vi "Simple Reader.vi"(8 "error in (no error)":errorcluster, 11 "Ocean Optics Driver in":refnum<class "Ocean Optics Driver.lvclass">) -> (0 "error out":errorcluster, 2 "Signals":dbl[](array[numeric]), 3 "Ocean Optics Driver out":refnum<class "Ocean Optics Driver.lvclass">)   [LabVIEW 2016, in "Ocean Optics Driver.lvclass"]
uses:
  Ocean Optics Driver.lvclass
  C:/github/NHMFL_Core/Libraries/Instruments/Instrument Driver/Instrument Driver.lvclass
  C:/github/NHMFL_Core/Libraries/Instruments/Spectrometer Driver/Spectrometer Driver.lvclass
  Instrument Driver/Instrument Driver.lvclass/Instrument Driver.ctl
  Spectrometer Driver/Spectrometer Driver.lvclass/Spectrometer Driver.ctl
  Instrument Driver/Write Channel names.vi
  Instrument Driver/Write Channel units.vi
  Spectrometer Driver/Read Peaks.vi
  Read Ocean optics configuration.vi
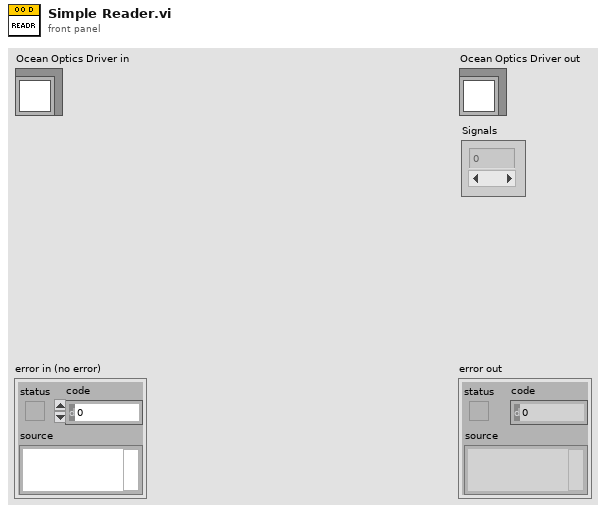
[diagram p1: front panel]
types:
  T1 = typedef "Peak Parameters.ctl" = cluster{"Amplitude":dbl, "Center":dbl, "Width":dbl}
  T2 = typedef "Ruby Spectra.lvclass/Ocean optics configuration.ctl" = cluster{"Integration time":dbl, "Fit parameters":T3, "Fit":bool, "Auto-update params":bool, "Save spectra":bool, "Reference wavelengh":dbl, "Background":path}
  T3 = typedef "Multi-peak Parameters.ctl" = cluster{"Function":enum16{"Gauss", "Lorentz"}, "Window width":dbl, "Initial guess":T1}
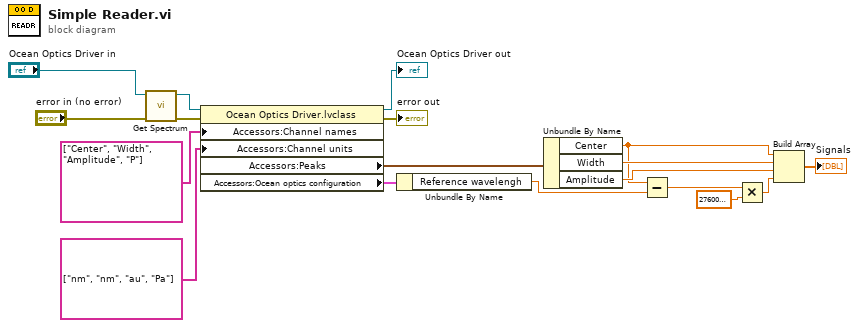
[diagram p0: block diagram]
diagram:
  n1 = call-dynamic "Get Spectrum.vi"("error in (no error)"="error in (no error)", "Ocean Optics Driver in"="Ocean Optics Driver in") -> ("error out"=w8:errorcluster, "Ocean Optics Driver out"=w15:refnum<class "Ocean Optics Driver.lvclass">)  [unwired: 7 in, 1 out]
  n2 = property class="Ocean Optics Driver.lvclass"(reference=w15, error in=w8, "Accessors:Channel names"=string[] ["Center", "Width", "Amplitude", "P"] ("Channel names"), "Accessors:Channel units"=string[] ["nm", "nm", "au", "Pa"] ("Channel names")) -> (reference out=→"Ocean Optics Driver out":refnum<class "Ocean Optics Driver.lvclass">, error out=→"error out":errorcluster, "Accessors:Peaks"=w7:T1, "Accessors:Ocean optics configuration"=w6:T2)
  n3 = Unbundle By Name(w6) -> ("Reference wavelengh"=w3:dbl)
  n4 = Unbundle By Name(w7) -> ("Center"=w2:dbl, "Width"=w14:dbl, "Amplitude"=w13:dbl)
  n5 = Subtract(x=w2, y=w3) -> (x-y=w5:dbl)
  n6 = Multiply(x=w5, y=2760000000.0) -> (x*y=w1:dbl)
  n7 = Build Array(w2, w14, w13, w1) -> (→"Signals":dbl[])
